vi "test visa.vi"() -> ()   [LabVIEW 2019]
panel:
  out "return count 2":u32
  out "read buffer":string
  in  "VISA resource name":refnum<visa-resource-name>
  out "return count":u32
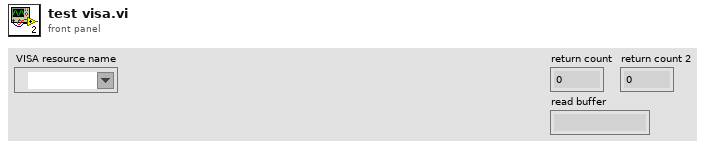
[diagram p1: front panel]
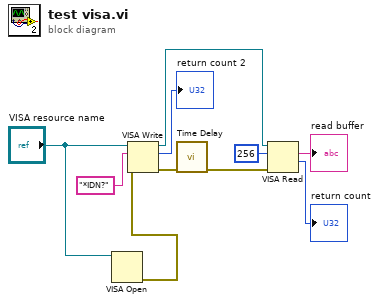
[diagram p0: block diagram]
diagram:
  n1 = VISA Open(VISA resource name="VISA resource name") -> (error out=w1:errorcluster)  [unwired: 4 in, 1 out]
  n2 = VISA Write(VISA resource name="VISA resource name", write buffer="*IDN?", error in (no error)=w1) -> (VISA resource name out=w9:refnum<visa-resource-name>, return count=→"return count 2":u32, error out=w10:errorcluster)
  n3 = call "Time Delay"("error in (no error)"=w10) -> ("error out"=w5:errorcluster)  [unwired: 10 in]
  n4 = VISA Read(VISA resource name=w9, byte count=u32 256, error in (no error)=w5) -> (read buffer=→"read buffer":string, return count=→"return count":u32)  [unwired: 2 out]
